vi "Configure Period Counter.vi"(8 "error in":errorcluster, 9 "Samples":i32=20 min=1 max=10000000, 11 "VISA resource name":refnum<visa-resource-name>) -> (0 "error out":errorcluster, 3 "VISA resource name out":refnum<visa-resource-name>)   [LabVIEW 2020, in "BDAQ-6104.lvlib"]
doc: "Configure the counter function on digital input pin 1."
uses:
  <instrlib>/BDAQ-6104/BDAQ-6104.lvlib
  <instrlib>/BDAQ-6104/Private/Edge Triger Type.ctl
panel:
  in  "Mode":T1=enum."FALLING"
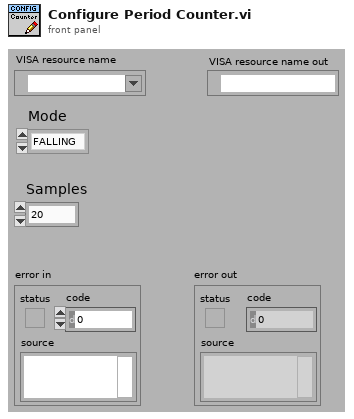
[diagram p1: front panel]
types:
  T1 = typedef "BDAQ-6104.lvlib/Edge Triger Type.ctl" = enum16{"CHANGE", "FALLING", "RISING"}
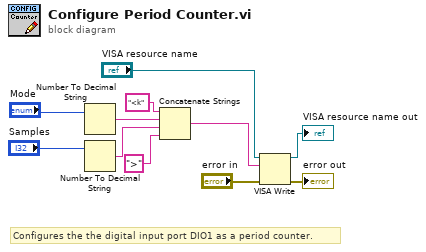
[diagram p0: block diagram]
diagram:
  # "Configures the the digital input port DIO1 as a period counter."
  n1 = Number To Decimal String(number="Mode") -> (decimal integer string=w10:string)  [unwired: 1 in]
  n2 = Number To Decimal String(number="Samples") -> (decimal integer string=w3:string)  [unwired: 1 in]
  n3 = Concatenate Strings("<k", w10, w3, ">") -> (w9:string)
  n4 = VISA Write(VISA resource name="VISA resource name", write buffer=w9, error in (no error)="error in") -> (VISA resource name out=→"VISA resource name out":refnum<visa-resource-name>, error out=→"error out":errorcluster)  [unwired: 1 out]
